vi "四段比较器（I8）.vi"(1 "输入数值":i8=20, 2 "低":i8=10, 3 "中":i8=50, 4 "高":i8=100) -> (0 "Range":enum16{"超低", "中偏低", "中偏高", "超高"}(ring)=enum."中偏低")   [LabVIEW 2011]
doc: "功能：\n\n返回一个枚举，表明输入数的范围，用于三段比较。\n\n\nCSXCS_366创建。"
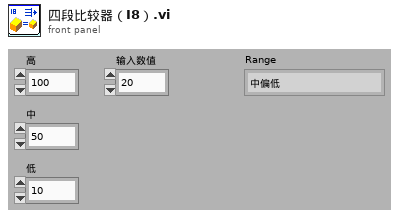
[diagram p1: front panel]
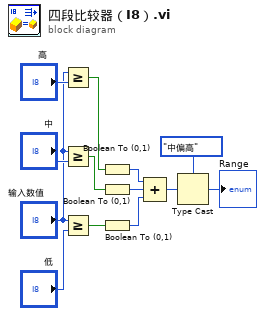
[diagram p0: block diagram]
diagram:
  n1 = Greater Or Equal?(x="输入数值", y="高") -> (x >= y?=w4:bool)
  n2 = Greater Or Equal?(x="输入数值", y="中") -> (x >= y?=w11:bool)
  n3 = Greater Or Equal?(x="输入数值", y="低") -> (x >= y?=w12:bool)
  n4 = Boolean To (0,1)(Boolean=w4) -> (0, 1=w1:i16)
  n5 = Boolean To (0,1)(Boolean=w11) -> (0, 1=w9:i16)
  n6 = Boolean To (0,1)(Boolean=w12) -> (0, 1=w10:i16)
  n7 = Compound Arithmetic op=ADD(w1, w9, w10) -> (w8:i16)
  n8 = Type Cast(type=enum16{"超低", "中偏低", "中偏高", "超高"}."中偏高" ("Range"), x=w8) -> (*(type *) &x=→"Range":enum16{"超低", "中偏低", "中偏高", "超高"})
